vi "Error Converter (ErrCode or Status).vi"(8 "error in (no error)":errorcluster, 10 "Language":T1 items=["System dependent", "Not available", "Not available", "Not available", "Not available", "Not available", "Not available", "Deutsch", "Not available", "English", "Español", "Not available", "Français", "Not available", "Not available", "Not available", "Italiano"], 11 "error code":i32) -> (0 "error out":errorcluster)   [LabVIEW 2020, in "PCANBasic.lvlib"]
uses:
  PCANBasic.lvlib
  Controls/Error language selector.ctl
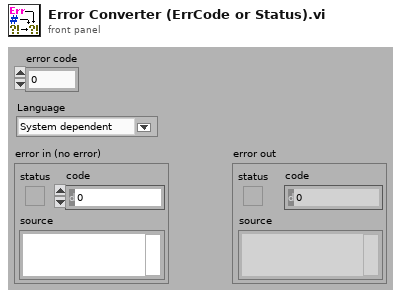
[diagram p1: front panel]
types:
  T1 = typedef "PCANBasic.lvlib/Error language selector.ctl" = u16
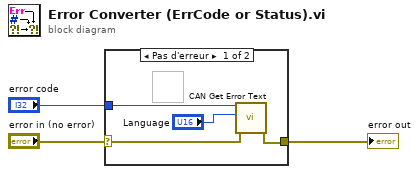
[diagram p0: block diagram]
diagram:
  n1 = case shown="Pas d'erreur" "error in (no error)" {
    selector: "error in (no error)" -> [w7 w8]
    tunnel: [w5 w8] -> w2
    tunnel: "error code" -> [w6 _]
    frame No Error {
      n2 = call "CAN Get Error Text.vi"("error in (no error)"=w7, "Language"="Language", "Error"=w6) -> ("error out"=w5:errorcluster)  [unwired: 8 in]
    }
    frame Error {
    }
  }
  "error out" <- w2
